vi "dsc9513SingleCounterControl.vi"(8 "error in":errorcluster, 9 "action":T1, 10 "counter":u8, 11 "board":i16) -> (0 "error out":errorcluster, 2 "counter_out":u8, 3 "boardOut":i16)   [LabVIEW 2011, in "Diamond Universal Driver.lvlib"]
doc: "Template for creating new DSC universal driver wrappers in Labview."
uses:
  Diamond Universal Driver.lvlib
  Controls/QMM ACTION.ctl
  Controls/error codes.ctl
  Instruments/WL OPC/Support/dlls/dscud.dll
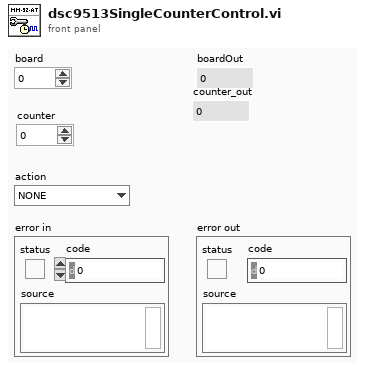
[diagram p1: front panel]
types:
  T1 = typedef "QMM ACTION.ctl" = enum8{"NONE", "ARM", "LOAD", "LOAD AND ARM", "DISARM AND SAVE", "SAVE", "DISARM"}
  T2 = typedef "Diamond Universal Driver.lvlib/error codes.ctl" = enum8{"DE_NONE", "DE_HW_FAILURE", "DE_SW_FAILURE", "DE_HW_NOT_SUPPORTED", "DE_SW_NOT_SUPPORTED", "DE_INVALID_PARM", "DE_ALTERNATE_IN_PROGRESS", "DE_NONE_IN_PROGRESS", "DE_BUFFER_ROLLOVER", "DE_INVALID_ERROR_CODE", "DE_ALREADY_PAUSED", "DE_OVERFLOW", "DE_INVALID_FUNC", "DE_DSCUDH_INVALID", "DE_INVALID_BOARD", "DE_BOARD_LIMIT_REACHED", "DE_BOARD_BUSY", "DE_INVALID_WINDRVR_HANDLE", "DE_INVALID_WINDRVR_VERSION", "DE_BAD_WINDRVR_BOARD_INIT", "DE_OPERATION_TIMED_OUT", "DE_INVALID_WINDRVR_KP", "DE_THREAD_FAILURE"}
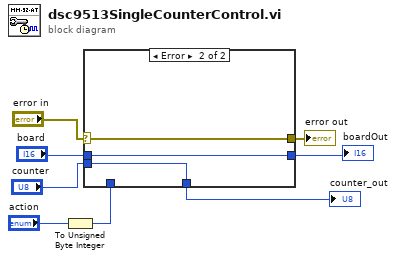
[diagram p0: block diagram]
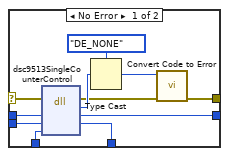
[diagram p2: hidden frame]
diagram:
  n1 = To Unsigned Byte Integer(number="action") -> (unsigned 8bit integer=w2:u8)
  n2 = case shown="Error" "error in" {
    selector: "error in" -> [w16 w22]
    tunnel: "board" -> [w14 w21]
    tunnel: [w13 w21] -> w6
    tunnel: [w12 w22] -> w5
    tunnel: "counter" -> [w11 w20]
    tunnel: w2 -> [w10 _]
    tunnel: [w9 w20] -> w1
    frame No Error {
      n3 = dll-call lib="C:/Users/mrichardson/Documents/Web Based Version Control SW/Instruments/WL OPC/Support/dlls/dscud.dll" fn="dsc9513SingleCounterControl"(error in=w16, "board"=w14, "counter"=w11, "action"=w10) -> (error out=w15:errorcluster, "error"=w17:u8, "board"=w13:i16, "counter"=w9:u8)  [unwired: 3 in, 1 out]
      n4 = Type Cast(type=error_codes."DE_NONE" ("error codes"), x=w17) -> (*(type *) &x=w19:T2)
      n5 = call "Convert Code to Error.vi"("error in"=w15, "error codes"=w19) -> ("error out"=w12:errorcluster)  [unwired: 9 in]
    }
    frame Error {
    }
  }
  "boardOut" <- w6
  "error out" <- w5
  "counter_out" <- w1
